vi "BuiltCurrentStateMsg.vi"(0 "State":T1 {"ILoad" format="%_6g"; "Fault Registers" format="%016x"; "VLoad" format="%_6g"; "VDCLink" format="%_6g"; "Detected Frequency" format="%1_6g"}, 11 "error in (no error)":errorcluster) -> (4 "CurrentStateMsg":refnum<class "JSON Object.lvclass">, 15 "error out":errorcluster)   [LabVIEW 2017, in "AppStateMachine runtime.lvclass"]
uses:
  AppStateMachine runtime.lvclass
  State.ctl
  StateId.ctl
  LED_Color.ctl
  <vilib>/NI/JSON Support for LabVIEW/JSON Data Classes/JSON Object/JSON Object.lvclass
  <vilib>/NI/JSON Support for LabVIEW/JSON Data Classes/JSON Object/New JSON Object (Empty).vi
  <vilib>/NI/JSON Support for LabVIEW/JSON Data Classes/JSON Object/Insert Key Value Pair (Single String).vi
  <vilib>/NI/JSON Support for LabVIEW/JSON Data Classes/JSON Object/Insert Key Value Pair (Single Boolean).vi
  <vilib>/NI/JSON Support for LabVIEW/JSON Data Classes/JSON Object/Insert Key Value Pair (Single Numeric).vi
  <vilib>/NI/JSON Support for LabVIEW/JSON Data Classes/JSON Helper/JSON Helper.lvclass
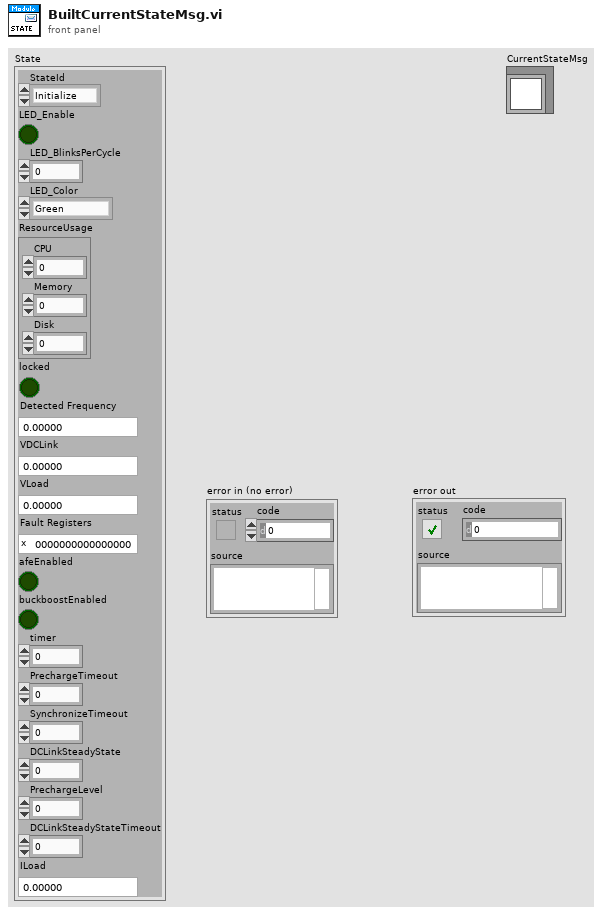
[diagram p1: front panel]
types:
  T1 = typedef "AppStateMachine runtime.lvclass/State.ctl" = cluster{"StateId":T2, "LED_Enable":bool, "LED_BlinksPerCycle":i32, "LED_Color":T3, "ResourceUsage":cluster{"CPU":dbl, "Memory":dbl, "Disk":dbl}, "locked":bool, "Detected Frequency":dbl, "VDCLink":dbl, "VLoad":dbl, "Fault Registers":u64, "afeEnabled":bool, "buckboostEnabled":bool, "timer":u32, "PrechargeTimeout":u32, "SynchronizeTimeout":u32, "DCLinkSteadyState":dbl, "PrechargeLevel":dbl, "DCLinkSteadyStateTimeout":u32, "ILoad":dbl}
  T2 = typedef "AppStateMachine runtime.lvclass/StateId.ctl" = enum16{"Initialize", "Idle", "TunePLL", "TuneAFE", "TuneBuckBoost", "Precharge", "Synchronize", "Ready", "EnableAFE", "EnableBuckBoost", "Powered", "SafeState", "UnrecoverableSafeState"}
  T3 = typedef "AppStateMachine runtime.lvclass/LED_Color.ctl" = enum16{"Green", "Yellow"}
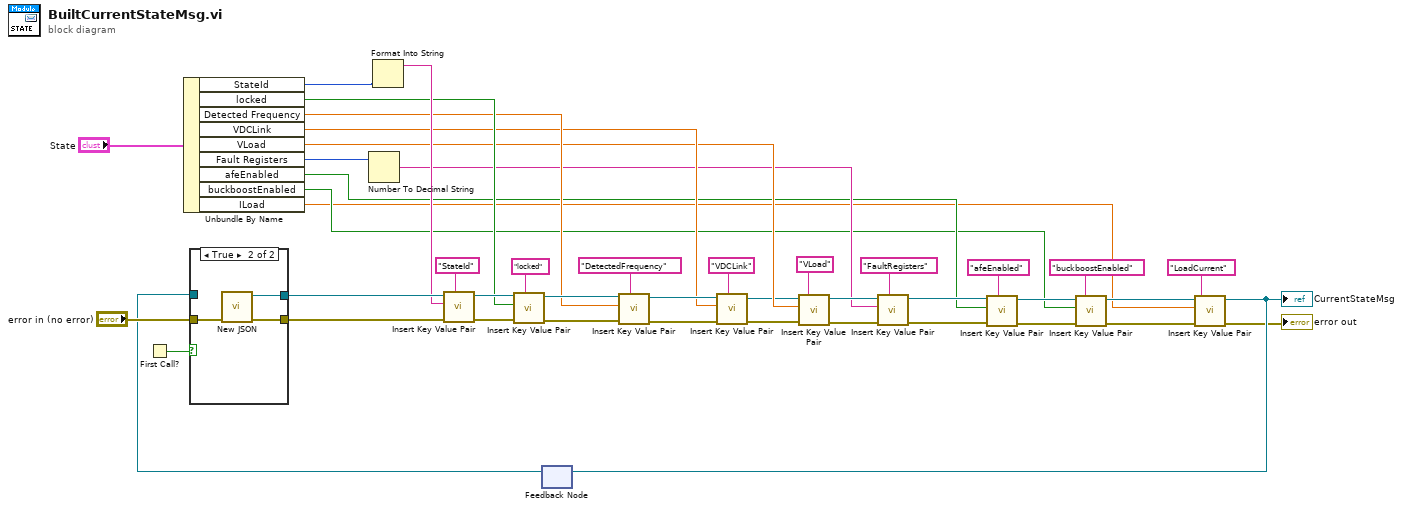
[diagram p0: block diagram]
diagram:
  n1 = First Call?() -> (First Call?: T/F=w41:bool)
  n2 = Unbundle By Name("State") -> ("StateId"=w44:T2, "locked"=w31:bool, "Detected Frequency"=w27:dbl, "VDCLink"=w23:dbl, "VLoad"=w20:dbl, "Fault Registers"=w39:u64, "afeEnabled"=w9:bool, "buckboostEnabled"=w8:bool, "ILoad"=w2:dbl)
  n3 = Number To Decimal String(number=w39) -> (decimal integer string=w15:string)  [unwired: 1 in]
  n4 = Format Into String(w44) -> (resulting string=w37:string)  [unwired: 3 in, 1 out]
  n5 = feedback #1() -> (w40:refnum<class "JSON Object.lvclass">)  [unwired: 1 in]
  n6 = case shown="True" w41 {
    tunnel: "error in (no error)" -> [w45 w49]
    tunnel: [w46 w48] -> w38
    tunnel: w40 -> [w46 _]
    tunnel: [w45 w47] -> w36
    frame False {
    }
    frame True {
      n7 = call-poly <vilib>:"New JSON.vi"("error in (no error)"=w49) -> ("error out"=w47:errorcluster, "JSON Object out"=w48:refnum<class "JSON Object.lvclass">)  [unwired: 9 in]
    }
  }
  n8 = call-poly <vilib>:"Insert Key Value Pair.vi"("key"="StateId", "error in (no error)"=w36, "value"=w37, "JSON Object in"=w38) -> ("error out"=w33:errorcluster, "JSON Object out"=w34:refnum<class "JSON Object.lvclass">)  [unwired: 5 in, 1 out]
  n9 = call-poly <vilib>:"Insert Key Value Pair.vi"("key"="locked", "error in (no error)"=w33, "value"=w31, "JSON Object in"=w34) -> ("error out"=w29:errorcluster, "JSON Object out"=w30:refnum<class "JSON Object.lvclass">)  [unwired: 5 in, 1 out]
  n10 = call-poly <vilib>:"Insert Key Value Pair.vi"("key"="DetectedFrequency", "error in (no error)"=w29, "value"=w27, "JSON Object in"=w30) -> ("error out"=w25:errorcluster, "JSON Object out"=w26:refnum<class "JSON Object.lvclass">)  [unwired: 5 in, 1 out]
  n11 = call-poly <vilib>:"Insert Key Value Pair.vi"("key"="VDCLink", "error in (no error)"=w25, "value"=w23, "JSON Object in"=w26) -> ("error out"=w22:errorcluster, "JSON Object out"=w19:refnum<class "JSON Object.lvclass">)  [unwired: 5 in, 1 out]
  n12 = call-poly <vilib>:"Insert Key Value Pair.vi"("key"="VLoad", "error in (no error)"=w22, "value"=w20, "JSON Object in"=w19) -> ("error out"=w17:errorcluster, "JSON Object out"=w18:refnum<class "JSON Object.lvclass">)  [unwired: 5 in, 1 out]
  n13 = call-poly <vilib>:"Insert Key Value Pair.vi"("key"="FaultRegisters", "error in (no error)"=w17, "value"=w15, "JSON Object in"=w18) -> ("error out"=w13:errorcluster, "JSON Object out"=w14:refnum<class "JSON Object.lvclass">)  [unwired: 5 in, 1 out]
  n14 = call-poly <vilib>:"Insert Key Value Pair.vi"("key"="afeEnabled", "error in (no error)"=w13, "value"=w9, "JSON Object in"=w14) -> ("error out"=w11:errorcluster, "JSON Object out"=w12:refnum<class "JSON Object.lvclass">)  [unwired: 5 in, 1 out]
  n15 = call-poly <vilib>:"Insert Key Value Pair.vi"("key"="buckboostEnabled", "error in (no error)"=w11, "value"=w8, "JSON Object in"=w12) -> ("error out"=w4:errorcluster, "JSON Object out"=w6:refnum<class "JSON Object.lvclass">)  [unwired: 5 in, 1 out]
  n16 = call-poly <vilib>:"Insert Key Value Pair.vi"("key"="LoadCurrent", "error in (no error)"=w4, "value"=w2, "JSON Object in"=w6) -> ("error out"=→"error out":errorcluster, "JSON Object out"=w5:refnum<class "JSON Object.lvclass">)  [unwired: 5 in, 1 out]
  "CurrentStateMsg" <- w5
  n17 = feedback-in #1(w5) -> ()
